vi "RunMe (Test Launcher Unit Test).vi"() -> ()   [LabVIEW 2013, in "Unit Tests for Runner.lvclass"]
uses:
  Unit Tests for Runner.lvclass
  classes/Test Runner/Test Runner.lvclass
panel:
  out "error out":errorcluster
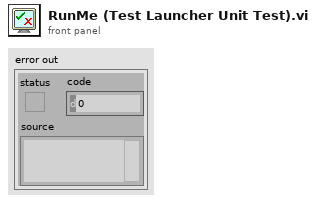
[diagram p1: front panel]
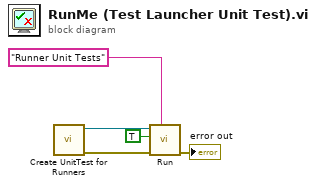
[diagram p0: block diagram]
diagram:
  n1 = call "Create UnitTest for Runners.vi"() -> ("error out"=w3:errorcluster, "Unit Tests for Runner out"=w4:refnum<class "Unit Tests for Runner.lvclass">)  [unwired: 10 in]
  n2 = call "Run.vi"("Name"="Runner Unit Tests", "error in (no error)"=w3, "Interactive"=TRUE, "Test Runner in"=w4) -> ("error out"=→"error out":errorcluster)  [unwired: 5 in, 2 out]
